vi "Action Init Trigger.vi"(0 "VISA resource name":refnum<visa-resource-name>, 2 "Inititiate Mode (1: Init Continuous)":i16(ring)=1 items=["Don't Initiate"=-1, "Initiate Single"=0, "Initiate Continuous"=1], 5 "error in (no error)":errorcluster) -> (14 "VISA resource name out":refnum<visa-resource-name>, 19 "error out":errorcluster)   [LabVIEW 2017, in "Keithley 2000.lvlib"]
doc: "This VI is used to initiate the trigger sequence of the instrument for single or continuous operation."
uses:
  Keithley 2000.lvlib
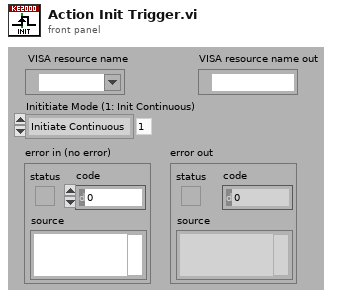
[diagram p1: front panel]
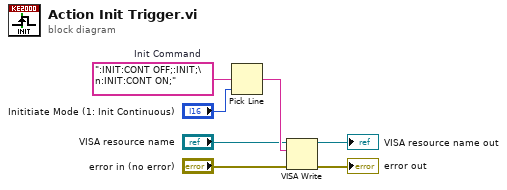
[diagram p0: block diagram]
diagram:
  w5 = ":INIT:CONT OFF;:INIT;\n:INIT:CONT ON;"  # Init Command
  n1 = Pick Line(multi-line string=w5, line index="Inititiate Mode (1: Init Continuous)") -> (output string=w3:string)  [unwired: 1 in]
  n2 = VISA Write(VISA resource name="VISA resource name", write buffer=w3, error in (no error)="error in (no error)") -> (VISA resource name out=→"VISA resource name out":refnum<visa-resource-name>, error out=→"error out":errorcluster)  [unwired: 1 out]
